vi "Actor Core.vi"(8 "error in":errorcluster, 11 "Nested in":refnum<class "MainUI Panel.lvclass">) -> (0 "error out":errorcluster, 3 "Actor out":refnum<class "Actor.lvclass">)   [LabVIEW 2019, in "MainUI.lvlib" / "MainUI Panel.lvlib" / "MainUI Panel.lvclass"]
doc: "(<B>Filename</B>: Actor Framework.lvlib:Actor.lvclass:Actor Core.vi)\n\nReceives messages to the actor, reacts to them, and initiates any error handling that may shut the actor down.\n\nDescendant classes may override this VI to append parallel tasks for the actor to complete while it handles messages. Overrides use the Call Parent Method node."
uses:
  MainUI Panel.lvclass
  C:/Program Files (x86)/National Instruments/LabVIEW 2019/vi.lib/ActorFramework/Actor/Actor.lvclass
  <vilib>/ActorFramework/Actor/Actor.lvclass
  <vilib>/Utility/miscctls.llb/LVPointTypeDef.ctl
  <vilib>/ActorFramework/Actor/Actor.lvclass/Actor.ctl
  <vilib>/ActorFramework/Message Enqueuer/Message Enqueuer.lvclass/Message Enqueuer.ctl
  MainUI Panel.lvclass/MainUI Panel.ctl
  <vilib>/Utility/miscctls.llb/LVPositionTypeDef.ctl
  <vilib>/ActorFramework/Message Enqueuer/Init from Existing Queue.vi
  <vilib>/ActorFramework/Message Enqueuer/Enqueue.vi
  <vilib>/ActorFramework/Stop Msg/Stop Msg.lvclass
  C:/Program Files (x86)/National Instruments/LabVIEW 2019/vi.lib/ActorFramework/Message/Message.lvclass
  <vilib>/ActorFramework/Message Priority Queue/Priority Enqueue.vi
  ModuleAbstract/ModuleAbstract.lvclass
  <vilib>/ActorFramework/Message Enqueuer/Message Enqueuer.lvclass
panel:
  out "LOGO":picture
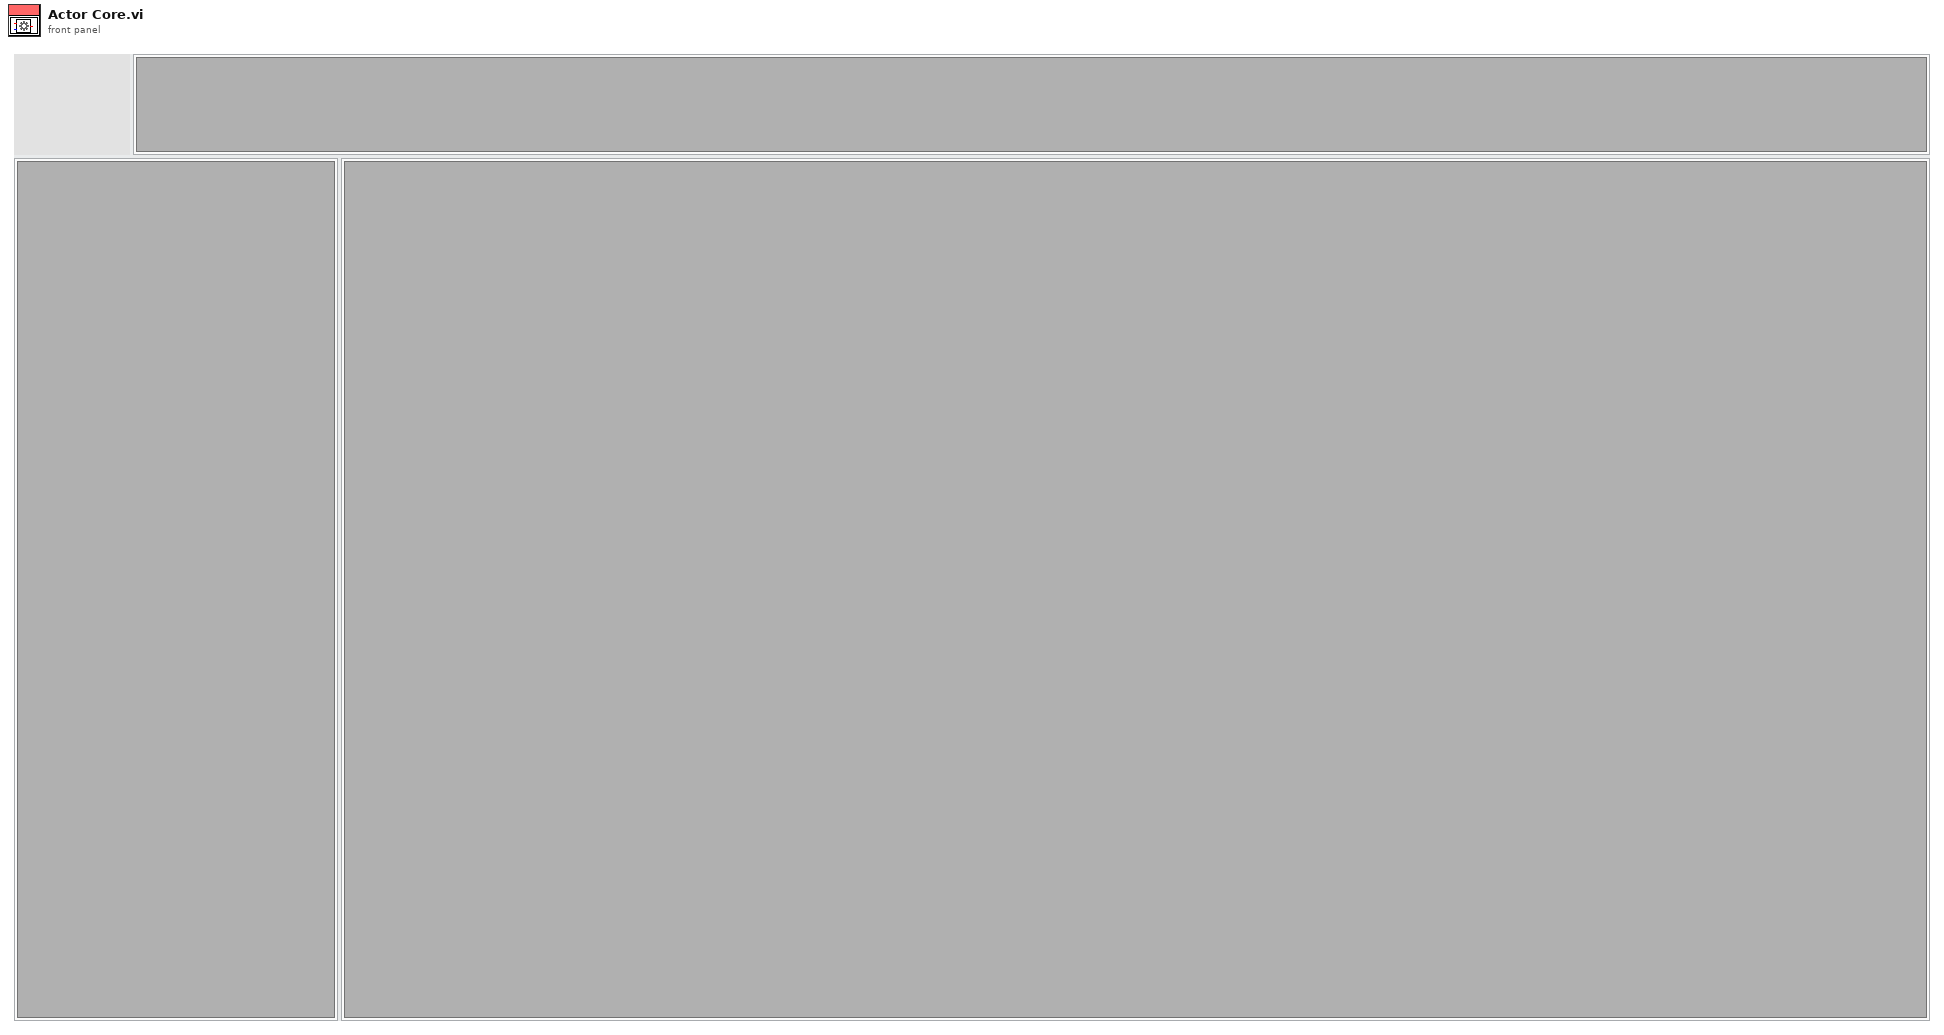
[diagram p1: front panel]
types:
  T1 = typedef "LVPointTypeDef.ctl" = cluster{"Horizontal":i16, "Vertical":i16}
  T2 = typedef "imagedata.ctl" = cluster{"image type":i32, "image depth":i32, "image":u8[], "mask":u8[], "colors":u32[], "Rectangle":cluster{"left":i16, "top":i16, "right":i16, "bottom":i16}}
  T3 = cluster{"Stop":refnum<user-event>, "LOGO":refnum<user-event>}
  T4 = typedef "LVPositionTypeDef.ctl" = cluster{"Left":i32, "Top":i32}
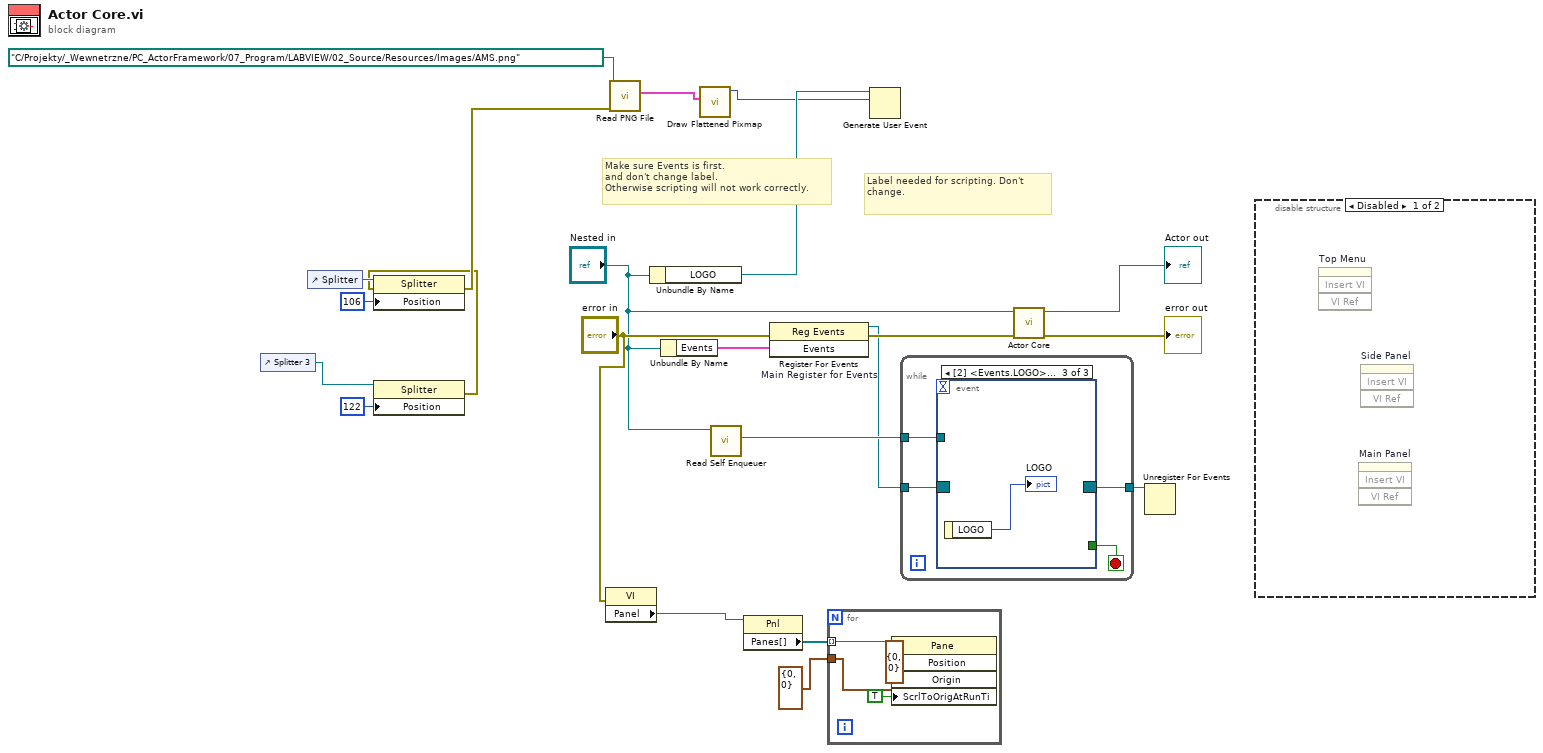
[diagram p0: block diagram]
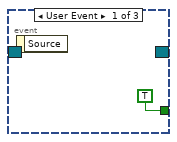
[diagram p3: hidden frame]
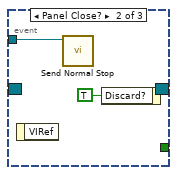
[diagram p4: hidden frame]
diagram:
  # "Label needed for scripting. Don't change."
  # "Make sure Events is first.\nand don't change label.\nOtherwise scripting will not work correctly."
  n1 = control-ref of="Splitter 3"() -> (w4:refnum<vi>)
  n2 = control-ref of="Splitter"() -> (w7:refnum<vi>)
  n3 = property class="Splitter"(reference=w4, "Position"=122 ("Splitter Position")) -> (error out=w2:errorcluster)  [unwired: 1 in, 1 out]
  n4 = property class="Splitter"(reference=w7, error in=w2, "Position"=106 ("Splitter Position")) -> (error out=w5:errorcluster)  [unwired: 1 out]
  n5 = property class="VI"(error in="error in") -> ("Panel"=w15:refnum<vi>)  [unwired: 1 in, 2 out]
  n6 = call <vilib>:"Read PNG File.vi"("error in (no error)"=w5, "path to PNG file"=path "C:/Projekty/_Wewnetrzne/PC_ActorFramework/07_Program/LABVIEW/02_Source/Resources/Images/AMS.png" ("Path")) -> ("image data"=w9:T2)  [unwired: 7 in, 2 out]
  n7 = Unbundle By Name("Nested in") -> ("LOGO"=w10:refnum<user-event>)
  n8 = Unbundle By Name("Nested in") -> ("Events"=w20:T3)
  n9 = call <vilib>:"Draw Flattened Pixmap.vi"("image data"=w9) -> ("new picture"=w8:picture)  [unwired: 8 in]
  n10 = call <vilib>:"Read Self Enqueuer.vi"("Actor"="Nested in") -> ("Self Enqueuer"=w18:refnum<class "Message Enqueuer.lvclass">)  [unwired: 10 in]
  n11 = property class="Pnl"(reference=w15) -> ("Panes[]"=w16:refnum<vi>[])  [unwired: 1 in, 2 out]
  n12 = register-events "Main Register for Events"(error in="error in", w20) -> (reference out=w12:refnum<event-registration>, error out=w17:errorcluster)  [unwired: 1 in]
  n13 = for {
    tunnel: w16 -> [w26] mode=indexing
    tunnel: T1 {"Horizontal"=0, "Vertical"=0} ("Origin") -> [w24]
    n14 = property class="Pane"(reference=w26, "Position"=T4 {"Left"=0, "Top"=0}, "Origin"=w24, "ScrlToOrigAtRunTi"=TRUE ("Scroll To Origin At Run Time")) -> ()  [unwired: 1 in, 2 out]
  }
  n15 = Generate User Event(user event=w10, event data cluster=w8) -> ()  [unwired: 2 in, 2 out]
  n16 = while {
    tunnel: w12 -> [w30]
    tunnel: [w28] -> w19
    tunnel: w18 -> [w27]
    stop <- w29 stop-if-true
    n17 = event "UI Events" shown="[2] <Events.LOGO>: User Event" {
      selector: w30 -> [_ _ _]
      dyn-events: [_ _ _] -> w28
      timeout: _ -> [_ _ _]
      tunnel: [TRUE _ _] -> w29
      tunnel: w27 -> [_ w32 _]
      event User Event {
        n18 = event-data() -> ()  [unwired: 1 in, 1 out]
      }
      event Panel Close? {
        n19 = event-data() -> ()  [unwired: 1 in, 1 out]
        n20 = call <vilib>:"Send Normal Stop.vi"("Message Enqueuer"=w32) -> ()  [unwired: 10 in, 1 out]
        n21 = event-data("Discard?"=TRUE) -> ()  [unwired: 1 in, 1 out]
      }
      event User Event {
        n22 = event-data() -> ("LOGO"=→"LOGO":picture)  [unwired: 1 in]
      }
    }
  }
  n23 = call-parent "Actor Core.vi"("error in"=w17, "Actor in"="Nested in") -> ("error out"=→"error out":errorcluster, "Actor out"=→"Actor out":refnum<class "Actor.lvclass">)  [unwired: 8 in]
  n24 = Unregister For Events(event registration refnum=w19) -> ()  [unwired: 1 in, 1 out]
  n25 = disable-structure shown="Disabled" {
    frame Disabled {
      n26 = invoke on="Top Menu" class="SubPnl" method="Insert VI"() -> ()  [unwired: 4 in, 4 out]
      n27 = invoke on="Main Panel" class="SubPnl" method="Insert VI"() -> ()  [unwired: 4 in, 4 out]
      n28 = invoke on="Side Panel" class="SubPnl" method="Insert VI"() -> ()  [unwired: 4 in, 4 out]
    }
    frame Enabled {
    }
  }
